vi "(SubVI) Set Camera Exposure Time.vi"(8 "error in (no error)":errorcluster, 10 "ExposureTime (us)":u32, 11 "Refnum in":T1) -> (0 "error out":errorcluster, 3 "Refnum out":T1)   [LabVIEW 2014]
uses:
  <vilib>/userdefined/High Color/IMAQdx.ctl
  <resource>/objmgr/imaqdx.rc
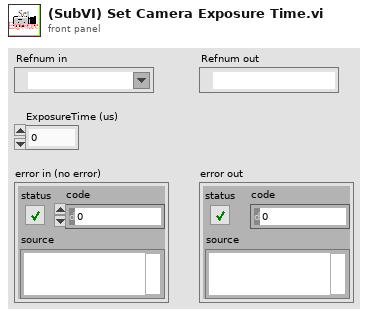
[diagram p1: front panel]
types:
  T1 = typedef "IMAQdx.ctl" = refnum<k21>
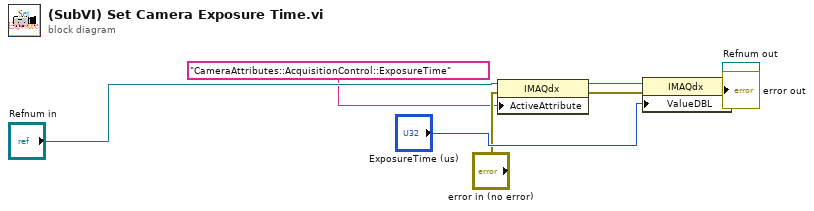
[diagram p0: block diagram]
diagram:
  n1 = property class="IMAQdx"(reference="Refnum in", error in="error in (no error)", "ActiveAttribute"="CameraAttributes::AcquisitionControl::ExposureTime") -> (reference out=w3:T1, error out=w6:errorcluster)
  n2 = property class="IMAQdx"(reference=w3, error in=w6, "ValueDBL"="ExposureTime (us)") -> (reference out=→"Refnum out":T1, error out=→"error out":errorcluster)
